vi "DAQ_photobleaching_pulse.vi"(2 "error in":errorcluster, 3 "physical channels":tag, 4 "Pulse length Ton (s)":dbl=0.025) -> (0 "error out":errorcluster)   [LabVIEW 2015]
uses:
  <vilib>/DAQmx/write.llb/DAQmx Write (Analog Wfm 1Chan NSamp).vi
  <vilib>/DAQmx/create/channels.llb/DAQmx Create Channel (AO-Voltage-Basic).vi
  <vilib>/DAQmx/configure/timing.llb/DAQmx Timing (Sample Clock).vi
  <vilib>/DAQmx/miscellaneous.llb/DAQmx Fill In Error Info.vi
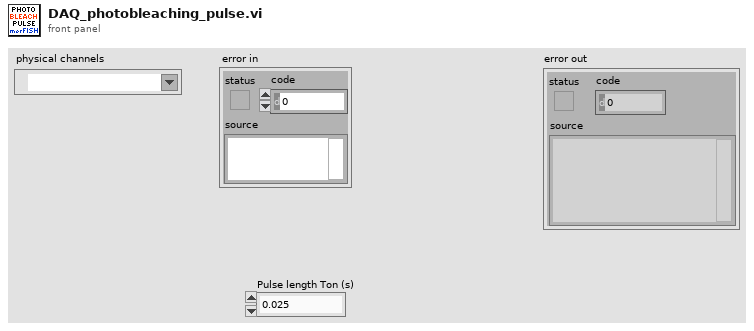
[diagram p1: front panel]
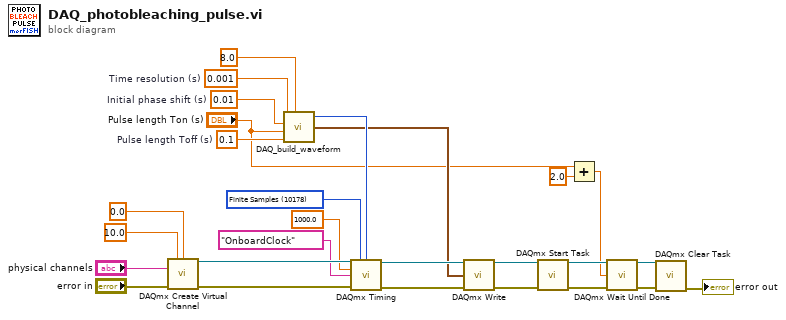
[diagram p0: block diagram]
diagram:
  w13 = 10178 items=["Finite Samples"=10178, "Continuous Samples"=10123, "Hardware Timed Single Point"=12522] ("sample mode")
  w24 = 0.1  # Pulse length Toff (s)
  w25 = 0.01  # Initial phase shift (s)
  w26 = 0.001  # Time resolution (s)
  n1 = call-poly <vilib>:"DAQmx Create Virtual Channel.vi"("maximum value"=10.0, "minimum value"=0.0, "physical channels"="physical channels", "error in"="error in") -> ("task out"=w21:refnum<k21>, "error out"=w20:errorcluster)  [unwired: 10 in]
  n2 = call "DAQ_build_waveform.vi"("Résolution temporelle"=w26, "Décalage"=w25, "Largeur impulsion"="Pulse length Ton (s)", "Remise à 0"=w24, "Pulse intensity"=8.0 ("y")) -> ("size(s)"=w19:i32, "waveform"=w16:waveform(dbl))  [unwired: 1 out]
  n3 = call-poly <vilib>:"DAQmx Timing.vi"("task/channels in"=w21, "sample mode"=w13, "samples per channel"=w19, "rate"=1000.0, "source"=tag "OnboardClock", "error in"=w20) -> ("task out"=w18:refnum<k21>, "error out"=w17:errorcluster)  [unwired: 8 in]
  n4 = call-poly <vilib>:"DAQmx Write.vi"("task/channels in"=w18, "data"=w16, "error in"=w17) -> ("task out"=w14:refnum<k21>, "error out"=w15:errorcluster)  [unwired: 10 in, 1 out]
  n5 = call <vilib>:"DAQmx Start Task.vi"("task/channels in"=w14, "error in"=w15) -> ("task out"=w9:refnum<k21>, "error out"=w10:errorcluster)  [unwired: 12 in]
  n6 = Add(x="Pulse length Ton (s)", y=2.0) -> (x+y=w2:dbl)
  n7 = call <vilib>:"DAQmx Wait Until Done.vi"("task/channels in"=w9, "timeout (sec)"=w2, "error in"=w10) -> ("task out"=w5:refnum<k21>, "error out"=w6:errorcluster)  [unwired: 11 in]
  n8 = call <vilib>:"DAQmx Clear Task.vi"("task in"=w5, "error in"=w6) -> ("error out"=→"error out":errorcluster)  [unwired: 13 in]
